vi "Joystick and Camera.vi"() -> ()   [LabVIEW 2020]
uses:
  Classes/Controller/Camera/Machine Vision.ctl
  Classes/Controller/I-O/I-O.lvclass
  Classes/Controller/Motion/Motion.lvclass
  Classes/Controller/Controller.lvclass
  Classes/Controller/Motion/A3200/A3200.lvclass
  Classes/Controller/Camera/Camera.lvclass
panel:
  in  "Machine Vision":T1
  in  "Z Go":bool
  in  "Position":dbl
  in  "XYZTheta":dbl[](array[numeric])
  in  "Go":bool
  in  "Joystick":bool
  out "Sum":dbl[](array[numeric])
  out "Gantry":dbl[](array[numeric])
  in  "Stop":bool
  out "Image":T2(plugin-control)
  out "Camera":dbl[](array[numeric])
  # "MOST CURRENT VERSION"
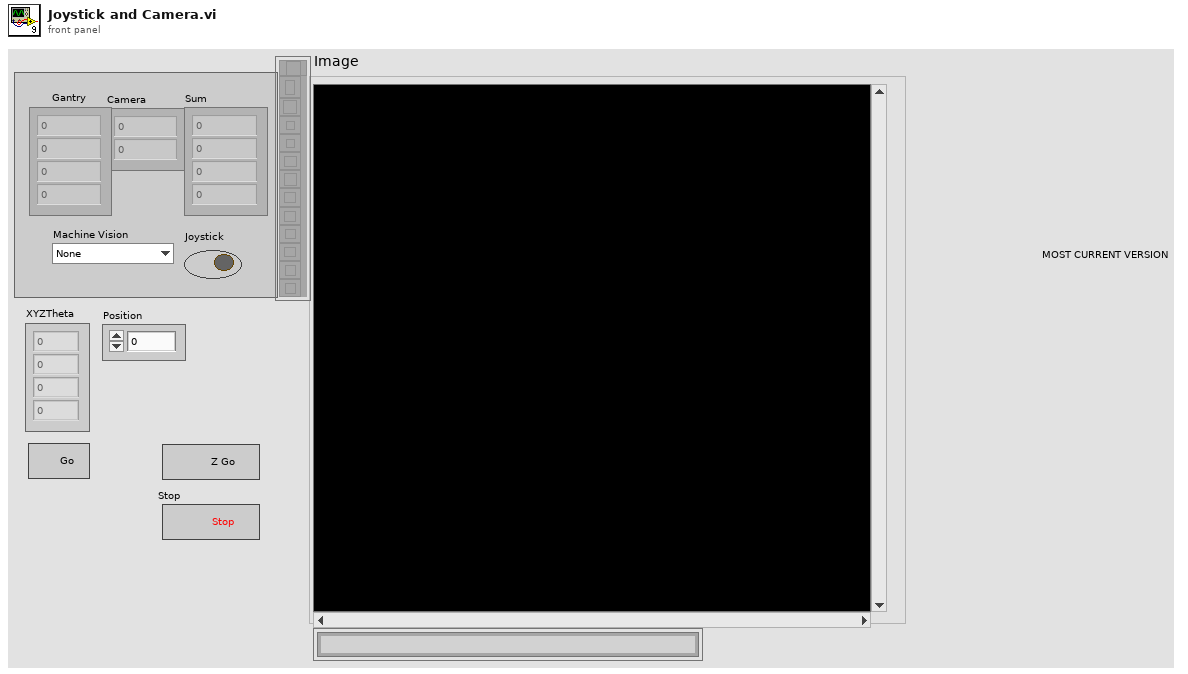
[diagram p1: front panel]
types:
  T1 = typedef "Camera.lvclass/Machine Vision.ctl" = enum16{"None", "Tray Fiducials", "HPK Silicon", "Hexaboard", "Corner (TL, BR)", "Corner (BL, TR)"}
  T2 = typedef "IMAQ Image.ctl" = refnum<image>
  T3 = typedef "Controller.lvclass/Controllers.ctl" = cluster{"I-O.lvclass":refnum<class "I-O.lvclass">, "Dispenser.lvclass":refnum<class "Dispenser.lvclass">, "Gantry":refnum<k24>}
  T4 = typedef "I-O.lvclass/Pin Map.ctl" = cluster{"Region Valves":i32[], "Extra Valves":dbl[][][], "Tool Primary Valve":i32, "Tool Secondary Valve":i32, "Region Sensors":i32[], "Extra Sensors":dbl[][][], "Tool Primary Sensor":dbl, "Tool Secondary Sensor":dbl, "Compression Sensor":dbl, "5V":i32}
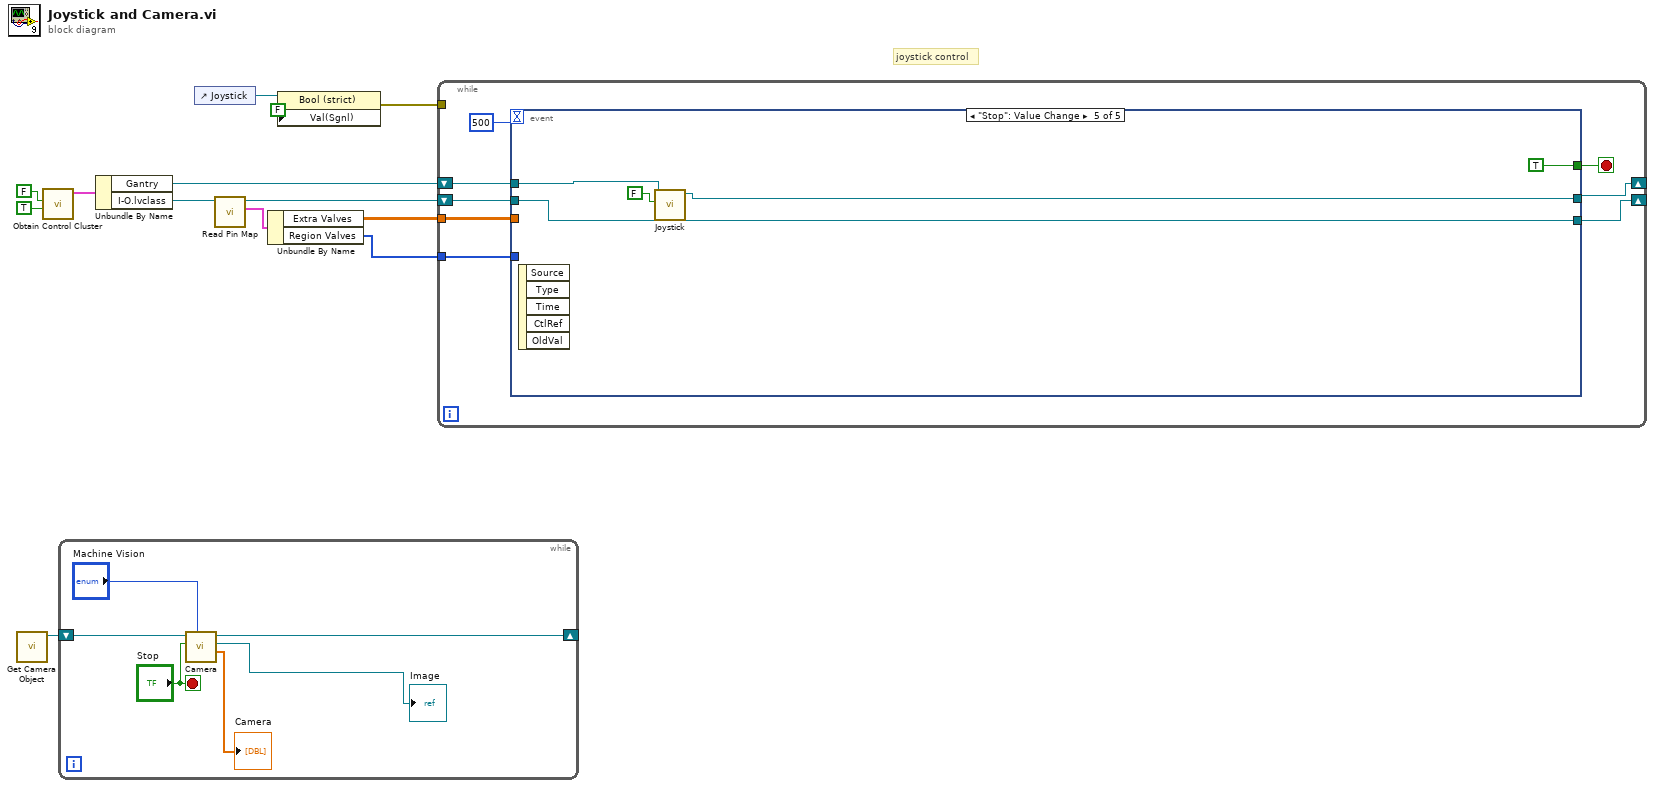
[diagram p0: block diagram]
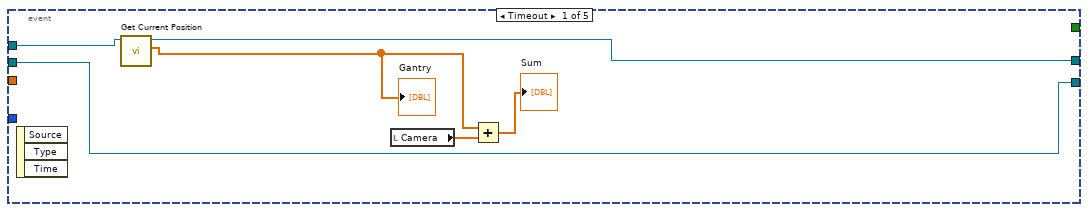
[diagram p2: hidden frame]
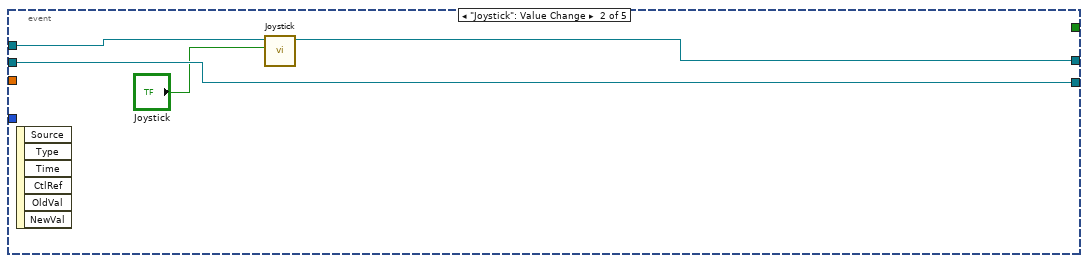
[diagram p3: hidden frame]
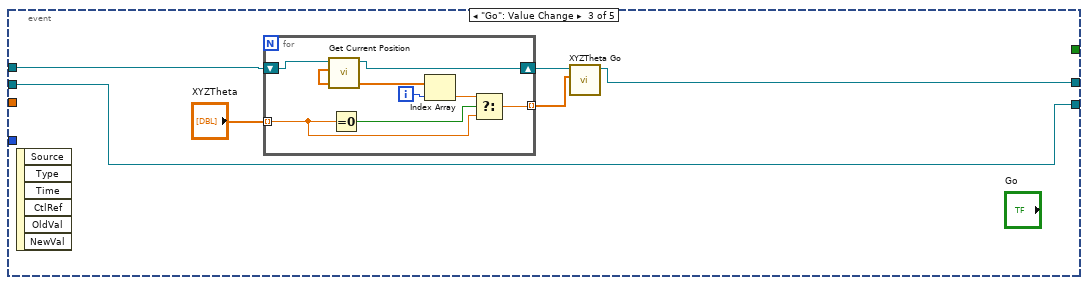
[diagram p4: hidden frame]
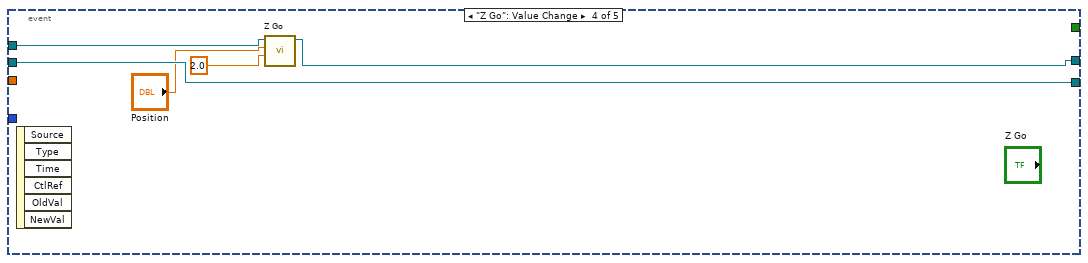
[diagram p5: hidden frame]
diagram:
  # "joystick control"
  n1 = call "Get Camera Object.vi"() -> ("Camera out"=w1:refnum<class "Camera.lvclass">)  [unwired: 10 in, 1 out]
  n2 = call "Obtain Control Cluster.vi"("I/O"=TRUE, "Dispense"=FALSE) -> ("Control Out"=w8:T3)  [unwired: 9 in]
  n3 = while {
    shift-right: [w18] -> _
    shift-left: w1 -> [w19]
    stop <- "Stop" stop-if-true
    n4 = call "Camera.vi"("Machine Vision"="Machine Vision", "Stop"="Stop", "Camera in"=w19) -> ("Camera"=→"Camera":dbl[], "Image"=→"Image":T2, "Camera out"=w18:refnum<class "Camera.lvclass">)  [unwired: 5 in, 1 out]
  }
  n5 = Unbundle By Name(w8) -> ("Gantry"=w7:refnum<k24>, "I-O.lvclass"=w6:refnum<class "I-O.lvclass">)
  n6 = control-ref of="Joystick"() -> (w12:refnum<vi>)
  n7 = call-dynamic "Read Pin Map.vi"("I-O in"=w6) -> ("Pin Map 2"=w4:T4, "I-O out"=w5:refnum<class "I-O.lvclass">)  [unwired: 8 in, 1 out]
  n8 = Unbundle By Name(w4) -> ("Extra Valves"=w2:dbl[][][], "Region Valves"=w3:i32[])
  n9 = property class="Bool (strict)"(reference=w12, "Val(Sgnl)"=FALSE ("Value (Signaling)")) -> (error out=w11:errorcluster)  [unwired: 1 in, 1 out]
  n10 = while {
    shift-right: [w20] -> _
    shift-left: w7 -> [w25]
    tunnel: w11 -> [_]
    shift-right: [w23] -> _
    shift-left: w5 -> [w24]
    tunnel: w3 -> [w22]
    tunnel: w2 -> [w21]
    stop <- w26 stop-if-true
    n11 = event shown="[4] \"Stop\": Value Change" {
      selector: _ -> [_ _ _ _ _]
      dyn-events: _ -> [_ _ _ _ _]
      timeout: 500 -> [_ _ _ _ _]
      tunnel: [_ _ _ _ TRUE] -> w26
      tunnel: w25 -> [w29 w34 w42 w55 w58]
      tunnel: w24 -> [w31 w37 w39 w56 w60]
      tunnel: [w31 w37 w39 w56 w60] -> w23
      tunnel: w22 -> [_ _ _ _ _]
      tunnel: w21 -> [_ _ _ _ _]
      tunnel: [w28 w35 w38 w52 w57] -> w20
      event Timeout {
        n12 = event-data() -> ()  [unwired: 1 in, 3 out]
        n13 = call "Get Current Position.vi"("Gantry 2"=w29) -> ("XYZTheta Out"=w30:dbl[], "Gantry 3"=w28:refnum<k24>)  [unwired: 8 in, 1 out]
        "Gantry" <- w30
        n14 = local read "Camera"() -> (w33:dbl[])
        n15 = Add(x=w30, y=w33) -> (x+y=→"Sum":dbl[])
      }
      event "Joystick": Value Change {
        n16 = event-data() -> ()  [unwired: 1 in, 6 out]
        n17 = call "Joystick.vi"("Joystick"="Joystick", "Gantry 2"=w34) -> ("Gantry 3"=w35:refnum<k24>)  [unwired: 8 in, 1 out]
      }
      event "Go": Value Change {
        n18 = event-data() -> ()  [unwired: 1 in, 6 out]
        n19 = for {
          tunnel: "XYZTheta" -> [w49] mode=indexing
          tunnel: [w47] -> w41 mode=indexing
          shift-right: [w44] -> w40
          shift-left: w42 -> [w45]
          i -> [w51]
          n20 = call "Get Current Position.vi"("Gantry 2"=w45) -> ("XYZTheta Out"=w46:dbl[], "Gantry 3"=w44:refnum<k24>)  [unwired: 8 in, 1 out]
          n21 = Equal To 0?(x=w49) -> (x = 0?=w50:bool)
          n22 = Index Array(array=w46, index=w51) -> (element=w48:dbl)
          n23 = Select(t=w48, s=w50, f=w49) -> (s? t:f=w47:dbl)
        }
        n24 = call "XYZTheta Go.vi"("XYZTheta In"=w41, "Gantry 2"=w40) -> ("Gantry 3"=w38:refnum<k24>)  [unwired: 7 in, 2 out]
      }
      event "Z Go": Value Change {
        n25 = event-data() -> ()  [unwired: 1 in, 6 out]
        n26 = call "Z Go.vi"("Speed"=2.0, "Position"="Position", "Gantry 2"=w55) -> ("Gantry 3"=w52:refnum<k24>)  [unwired: 7 in, 1 out]
      }
      event "Stop": Value Change {
        n27 = event-data() -> ()  [unwired: 1 in, 5 out]
        n28 = call "Joystick.vi"("Joystick"=FALSE, "Gantry 2"=w58) -> ("Gantry 3"=w57:refnum<k24>)  [unwired: 8 in, 1 out]
      }
    }
  }
